vi "CLSUIP_CalculateFutureParent.vi"(8 "error in (no error)":errorcluster, 11 "VIRetooler in":refnum<class "VIRetooler.lvclass">) -> (0 "error out":errorcluster, 2 "NewParentItem":refnum<vi>, 3 "VIRetooler out":refnum<class "VIRetooler.lvclass">)   [LabVIEW 2021, in "MemberVICreation.lvlib" / "VIRetooler.lvclass"]
uses:
  <resource>/Framework/Providers/LVClassLibrary/NewAccessors/VIRetooler/VIRetooler.lvclass
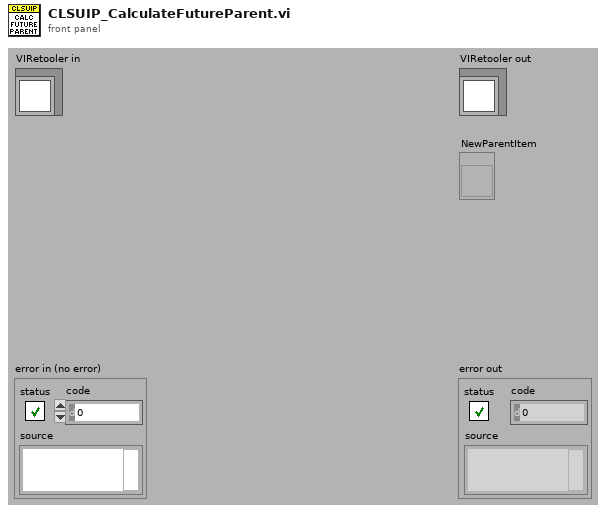
[diagram p1: front panel]
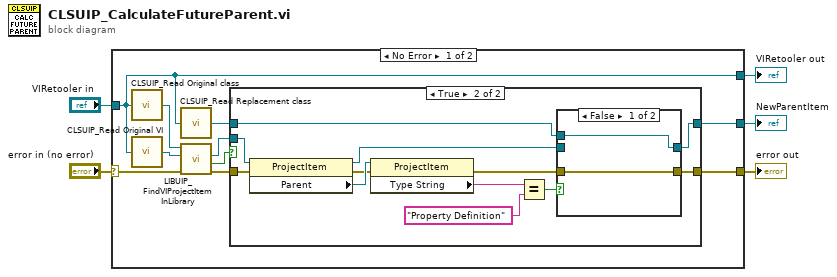
[diagram p0: block diagram]
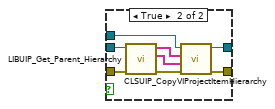
[diagram p3: hidden frame]
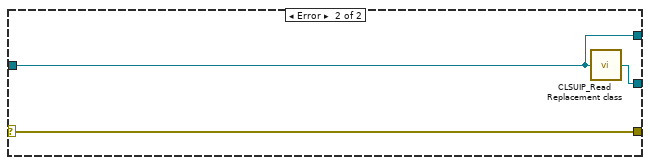
[diagram p4: hidden frame]
diagram:
  n1 = case shown="No Error" "error in (no error)" {
    selector: "error in (no error)" -> [w14 w42]
    tunnel: [w11 w42] -> w4
    tunnel: [w6 w41] -> w2
    tunnel: "VIRetooler in" -> [w6 w41]
    tunnel: [w10 w40] -> w1
    frame No Error {
      n2 = call <resource>:"CLSUIP_Read Original class.vi"("VIRetooler.lvclass in"=w6) -> ("Orig class"=w8:refnum<vi>)
      n3 = call <resource>:"CLSUIP_Read Original VI.vi"("VIRetooler.lvclass in"=w6) -> ("Original VI"=w15:refnum<vi>)
      n4 = call <resource>:"CLSUIP_Read Replacement class.vi"("VIRetooler.lvclass in"=w6) -> ("Replacement class"=w7:refnum<vi>)
      n5 = call <resource>:"LIBUIP_FindVIProjectItemInLibrary.vi"("error in (no error)"=w14, "VI Refnum"=w15, "Project Item"=w8) -> ("error out"=w13:errorcluster, "Found?"=w9:bool, "Project Item out"=w12:refnum<vi>)  [unwired: 5 in, 1 out]
      n6 = case shown="True" w9 {
        tunnel: w13 -> [w17 w21]
        tunnel: w12 -> [_ w23]
        tunnel: [w17 w26] -> w11
        tunnel: [w16 w25] -> w10
        tunnel: w7 -> [w16 w18]
        frame False {
        }
        frame True {
          n7 = property class="ProjectItem"(reference=w23, error in=w21) -> (reference out=w22:refnum<vi>, error out=w20:errorcluster, "Parent"=w29:refnum<vi>)
          n8 = property class="ProjectItem"(reference=w29, error in=w20) -> (error out=w19:errorcluster, "Type String"=w28:string)  [unwired: 1 out]
          n9 = Equal?(x=w28, y="Property Definition") -> (x = y?=w24:bool)
          n10 = case shown="False" w24 {
            tunnel: w19 -> [w31 w39]
            tunnel: w22 -> [_ w38]
            tunnel: [w31 w34] -> w26
            tunnel: [w30 w33] -> w25
            tunnel: w18 -> [w30 w32]
            frame False {
            }
            frame True {
              n11 = call <resource>:"LIBUIP_Get_Parent_Hierarchy.vi"("error in"=w39, "Project Item in"=w38) -> ("error out"=w37:errorcluster, "Parent Types"=w35:string[], "Parent Names"=w36:string[])  [unwired: 7 in]
              n12 = call <resource>:"CLSUIP_CopyVIProjectItemHierarchy.vi"("error in"=w37, "Parent Types"=w35, "Parent Names"=w36, "StartingProjectItem"=w32) -> ("error out"=w34:errorcluster, "NewParentItem"=w33:refnum<vi>)  [unwired: 6 in]
            }
          }
        }
      }
    }
    frame Error {
      n13 = call <resource>:"CLSUIP_Read Replacement class.vi"("VIRetooler.lvclass in"=w41) -> ("Replacement class"=w40:refnum<vi>)
    }
  }
  "error out" <- w4
  "VIRetooler out" <- w2
  "NewParentItem" <- w1
